vi "get file siz.vi"() -> ()   [LabVIEW 2012, in "DAQOrcaFlash.lvclass"]
uses:
  DAQOrcaFlash.lvclass
panel:
  out "size (in bytes)":i64
  in  "file":path
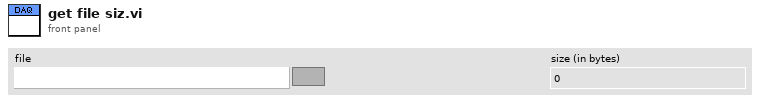
[diagram p1: front panel]
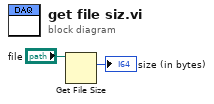
[diagram p0: block diagram]
diagram:
  n1 = Get File Size(file="file") -> (size (in bytes)=→"size (in bytes)":i64)  [unwired: 1 in, 2 out]
